vi "State_Machine.vi"(8 "error in (no error)":errorcluster caption="entrée d'erreur (pas d'erreur)", 11 "P1833_Access_Code.lvclass":refnum<class "P1833_Access_Code.lvclass">) -> (0 "error out":errorcluster caption="sortie d'erreur", 2 "Json_String":string, 3 "P1833_Access_Code.lvclass":refnum<class "P1833_Access_Code.lvclass">)   [LabVIEW 2020, in "Library Test.lvlib" / "P1833_Access_Code.lvclass"]
uses:
  P1833_Access_Code.lvclass
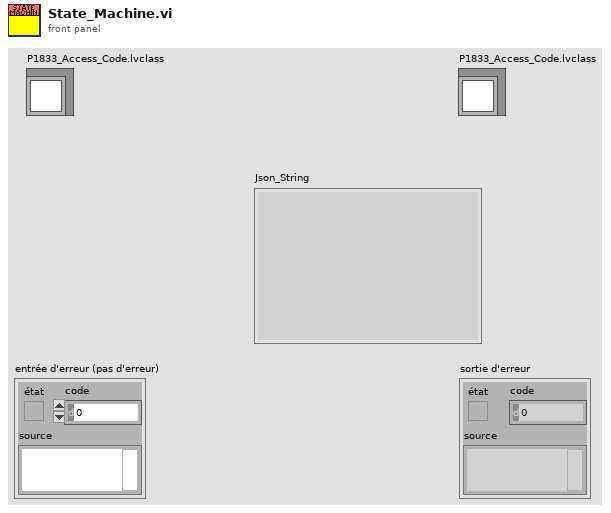
[diagram p1: front panel]
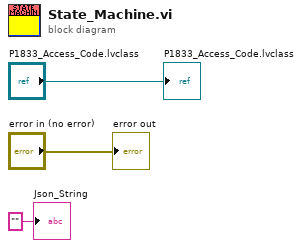
[diagram p0: block diagram]
diagram:
  "error out" <- "error in (no error)"
  "P1833_Access_Code.lvclass" <- "P1833_Access_Code.lvclass"
  "Json_String" <- "" ("Json_String")
